vi "get_statistics.vi"(8 "error in":errorcluster, 11 "all in one package in":T1={"memory structure"={"length of metadata [byte]"=5, "length of page [byte]"=2048, "length of measurement data on page [byte]"=2028, "length of dataset [byte]"=6}, "actigraph settings"={"sampling frequency [Hz]"=0.0, "measurement interval [± g]"=0, "high precision?"=FALSE, "number of pages"=0, "rate code"=0, "range code"=0, "id"=0}, "time informations"={"starting time"=timestamp(0 s since 1904-01-01), "ending time"=timestamp(0 s since 1904-01-01), "dt[s]"=0.0, "sampling rate [Hz]"=0.0, "length"=0.0}, "measurement data"={"number of samples per axis"=0, "timestamp array"=[], "offset array"=[], "x, y, z axis data"=[], "normalised magnitude of acceleartion vectors"={"t0"=timestamp(0 s since 1904-01-01), "dt"=1.0, "Y"=[]}, "calibration coefficients"={"Sx"=0.0, "Ox"=0.0, "Sy"=0.0, "Oy"=0.0, "Sz"=0.0, "Oz"=0.0}, "statistics"={"mean of x axis acceleration"=0.0, "standard devation of x axis acceleration"=0.0, "mean of y axis acceleration"=0.0, "standard devation of y axis acceleration"=0.0, "mean of z axis acceleration"=0.0, "standard devation of z axis acceleration"=0.0, "mean of normalised magnitude of acceleration"=0.0, "standard devation of normalised magnitude of acceleration"=0.0}, "battery voltage"={"t0"=timestamp(0 s since 1904-01-01), "dt"=1.0, "Y"=[]}, "magnitude of acceleartion vectors"={"t0"=timestamp(0 s since 1904-01-01), "dt"=1.0, "Y"=[]}}} {"measurement data"."calibration coefficients"."Oz" format="%#_12g"; "measurement data"."calibration coefficients"."Sz" format="%#_12g"; "measurement data"."calibration coefficients"."Oy" format="%#_12g"; "measurement data"."calibration coefficients"."Sy" format="%#_12g"; "measurement data"."calibration coefficients"."Ox" format="%#_12g"; "measurement data"."calibration coefficients"."Sx" format="%#_12g"; "time informations"."length" format="%<%H:%M:%S%3u>t"; "actigraph settings"."id" format="%02d"; "actigraph settings"."range code" format="%02x"; "actigraph settings"."rate code" format="%02x"}) -> (0 "error out":errorcluster, 3 "all in one package out":T1={"memory structure"={"length of metadata [byte]"=5, "length of page [byte]"=2048, "length of measurement data on page [byte]"=2028, "length of dataset [byte]"=6}, "actigraph settings"={"sampling frequency [Hz]"=0.0, "measurement interval [± g]"=0, "high precision?"=FALSE, "number of pages"=0, "rate code"=0, "range code"=0, "id"=0}, "time informations"={"starting time"=timestamp(0 s since 1904-01-01), "ending time"=timestamp(0 s since 1904-01-01), "dt[s]"=0.0, "sampling rate [Hz]"=0.0, "length"=0.0}, "measurement data"={"number of samples per axis"=0, "timestamp array"=[], "offset array"=[], "x, y, z axis data"=[], "normalised magnitude of acceleartion vectors"={"t0"=timestamp(0 s since 1904-01-01), "dt"=1.0, "Y"=[]}, "calibration coefficients"={"Sx"=0.0, "Ox"=0.0, "Sy"=0.0, "Oy"=0.0, "Sz"=0.0, "Oz"=0.0}, "statistics"={"mean of x axis acceleration"=0.0, "standard devation of x axis acceleration"=0.0, "mean of y axis acceleration"=0.0, "standard devation of y axis acceleration"=0.0, "mean of z axis acceleration"=0.0, "standard devation of z axis acceleration"=0.0, "mean of normalised magnitude of acceleration"=0.0, "standard devation of normalised magnitude of acceleration"=0.0}, "battery voltage"={"t0"=timestamp(0 s since 1904-01-01), "dt"=1.0, "Y"=[]}, "magnitude of acceleartion vectors"={"t0"=timestamp(0 s since 1904-01-01), "dt"=1.0, "Y"=[]}}} {"measurement data"."calibration coefficients"."Oz" format="%#_12g"; "measurement data"."calibration coefficients"."Sz" format="%#_12g"; "measurement data"."calibration coefficients"."Oy" format="%#_12g"; "measurement data"."calibration coefficients"."Sy" format="%#_12g"; "measurement data"."calibration coefficients"."Ox" format="%#_12g"; "measurement data"."calibration coefficients"."Sx" format="%#_12g"; "time informations"."length" format="%<%H:%M:%S%3u>t"; "actigraph settings"."id" format="%02d"; "actigraph settings"."range code" format="%02x"; "actigraph settings"."rate code" format="%02x"})   [LabVIEW 2020]
uses:
  Controls/control_all_in_one_package.ctl
  Controls/control_memory_structure.ctl
  Controls/control_measurement_settings.ctl
  Controls/control_time_informations.ctl
  Controls/control_measurement_data.ctl
  Controls/control_calibration_coefficients.ctl
  Controls/control_statistics.ctl
  <vilib>/Analysis/NI_AALBase.lvlib
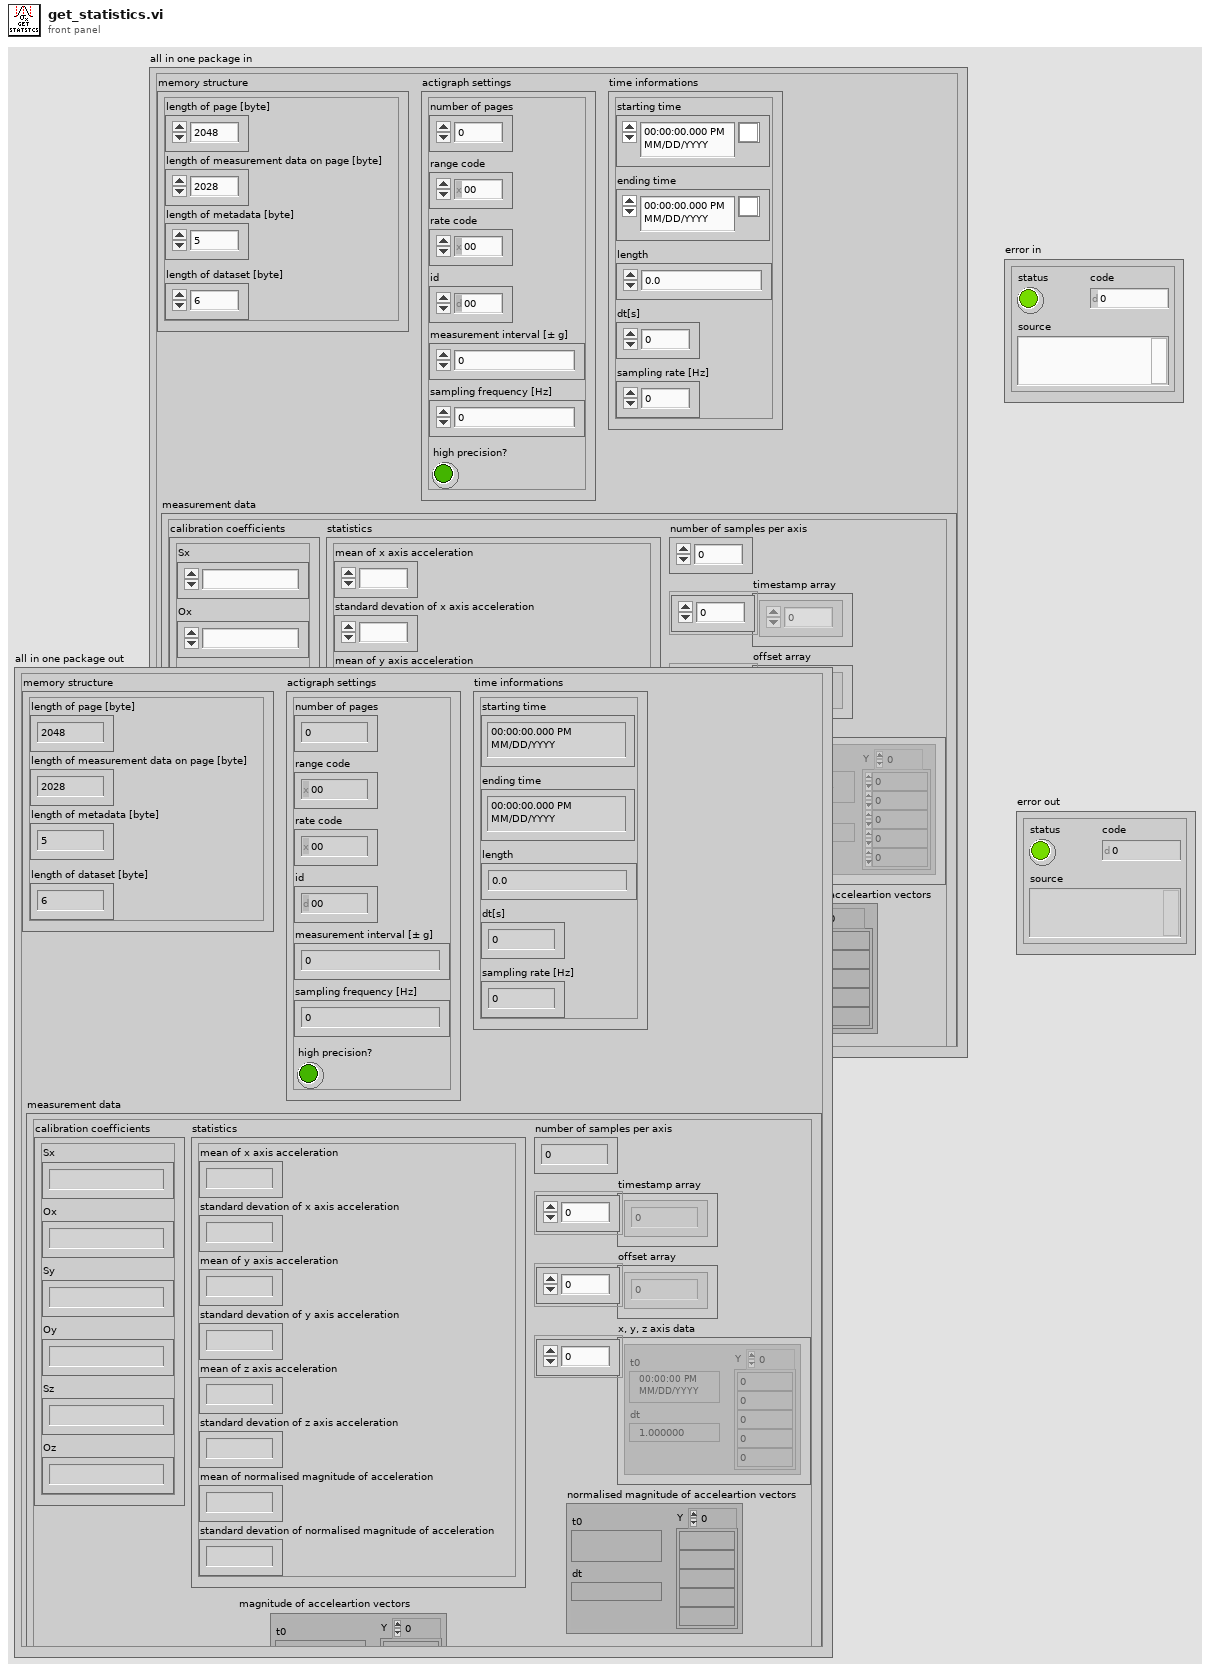
[diagram p1: front panel]
types:
  T1 = typedef "control_all_in_one_package.ctl" = cluster{"memory structure":T2, "actigraph settings":T3, "time informations":T4, "measurement data":T5}
  T2 = typedef "control_memory_structure.ctl" = cluster{"length of metadata [byte]":i32, "length of page [byte]":i32, "length of measurement data on page [byte]":i32, "length of dataset [byte]":i32}
  T3 = typedef "control_measurement_settings.ctl" = cluster{"sampling frequency [Hz]":dbl, "measurement interval [± g]":i32, "high precision?":bool, "number of pages":i32, "rate code":i32, "range code":i32, "id":i32}
  T4 = typedef "control_time_informations.ctl" = cluster{"starting time":timestamp, "ending time":timestamp, "dt[s]":dbl, "sampling rate [Hz]":dbl, "length":dbl}
  T5 = typedef "control_measurement_data.ctl" = cluster{"number of samples per axis":i32, "timestamp array":dbl[], "offset array":dbl[], "x, y, z axis data":waveform(dbl)[], "normalised magnitude of acceleartion vectors":waveform(dbl), "calibration coefficients":T6, "statistics":T7, "battery voltage":waveform(dbl), "magnitude of acceleartion vectors":waveform(dbl)}
  T6 = typedef "control_calibration_coefficients.ctl" = cluster{"Sx":dbl, "Ox":dbl, "Sy":dbl, "Oy":dbl, "Sz":dbl, "Oz":dbl}
  T7 = typedef "control_statistics.ctl" = cluster{"mean of x axis acceleration":dbl, "standard devation of x axis acceleration":dbl, "mean of y axis acceleration":dbl, "standard devation of y axis acceleration":dbl, "mean of z axis acceleration":dbl, "standard devation of z axis acceleration":dbl, "mean of normalised magnitude of acceleration":dbl, "standard devation of normalised magnitude of acceleration":dbl}
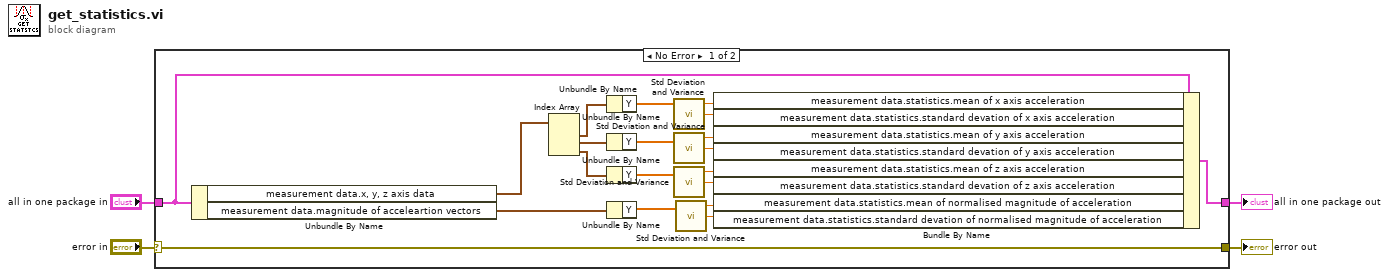
[diagram p0: block diagram]
diagram:
  n1 = case shown="No Error" "error in" {
    selector: "error in" -> [w24 w25]
    tunnel: [w24 w25] -> w3
    tunnel: "all in one package in" -> [w16 w26]
    tunnel: [w15 w26] -> w1
    frame No Error {
      n2 = Unbundle By Name(w16) -> ("measurement data.x, y, z axis data"=w23:waveform(dbl)[], "measurement data.magnitude of acceleartion vectors"=w17:waveform(dbl))
      n3 = Index Array(array=w23) -> (element #1=w22:waveform(dbl), element #2=w21:waveform(dbl), element #3=w20:waveform(dbl))  [unwired: 3 in]
      n4 = Unbundle By Name(w22) -> ("Y"=w19:dbl[])
      n5 = Unbundle By Name(w21) -> ("Y"=w18:dbl[])
      n6 = Unbundle By Name(w20) -> ("Y"=w6:dbl[])
      n7 = Unbundle By Name(w17) -> ("Y"=w5:dbl[])
      n8 = call <vilib>:"Std Deviation and Variance.vi"("X"=w19) -> ("mean"=w14:dbl, "standard deviation"=w13:dbl)  [unwired: 1 in, 1 out]
      n9 = call <vilib>:"Std Deviation and Variance.vi"("X"=w18) -> ("mean"=w12:dbl, "standard deviation"=w11:dbl)  [unwired: 1 in, 1 out]
      n10 = call <vilib>:"Std Deviation and Variance.vi"("X"=w6) -> ("mean"=w10:dbl, "standard deviation"=w9:dbl)  [unwired: 1 in, 1 out]
      n11 = call <vilib>:"Std Deviation and Variance.vi"("X"=w5) -> ("mean"=w8:dbl, "standard deviation"=w7:dbl)  [unwired: 1 in, 1 out]
      n12 = Bundle By Name(cluster=w16, "measurement data.statistics.mean of x axis acceleration"=w14, "measurement data.statistics.standard devation of x axis acceleration"=w13, "measurement data.statistics.mean of y axis acceleration"=w12, "measurement data.statistics.standard devation of y axis acceleration"=w11, "measurement data.statistics.mean of z axis acceleration"=w10, "measurement data.statistics.standard devation of z axis acceleration"=w9, "measurement data.statistics.mean of normalised magnitude of acceleration"=w8, "measurement data.statistics.standard devation of normalised magnitude of acceleration"=w7) -> (w15:T1)
    }
    frame Error {
    }
  }
  "error out" <- w3
  "all in one package out" <- w1
